vi "DSP_conditioning_Tx.vi"(1 "reset":bool, 4 "tx.frequency shift":fxp<+/-,48,0>, 5 "IQ data":T1, 6 "tx.phase":fxp<+/-,21,0>, 7 "input valid":bool, 8 "tx.delay":fxp<+/-,18,0>, 9 "tx.impairments":T3, 10 "tx.input sample rate":fxp<+,48,1>, 11 "tx.gain":T2) -> (0 "tx.dsp reset done":bool, 2 "output valid":bool, 3 "data out":T1)   [LabVIEW 2017]
uses:
  <instrlib>/_niInstr/DSP/v1/Shared/Public/IQ Impairments.ctl
  <instrlib>/_niInstr/DSP/v1/Shared/Public/IQ Gain.ctl
  <instrlib>/_niInstr/DSP/v1/Shared/Public/IQ Data.ctl
  <instrlib>/_niInstr/DSP/v1/FPGA/Public/Sub VIs/Digital Gain/Digital Gain - 1 spc.vi
  <instrlib>/_niInstr/DSP/v1/FPGA/Public/Sub VIs/Frequency Shift/Frequency Shift - 1 spc.vi
  <instrlib>/_niInstr/DSP/v1/FPGA/Public/Sub VIs/IQ Impairments/IQ Impairments - 1 spc.vi
  <instrlib>/_niInstr/DSP/v1/FPGA/niInstr DSP v1 FPGA.lvlib
  <instrlib>/_niInstr/Basic Elements/v1/FPGA/niInstr Basic Elements v1 FPGA.lvlib
  <instrlib>/_niInstr/DSP/v1/FPGA/Public/Sub VIs/Fractional Interpolator/Fractional Interpolator - 1 spc - 2x oc.vi
  <instrlib>/_niInstr/DSP/v1/Shared/niInstr DSP v1 Shared.lvlib
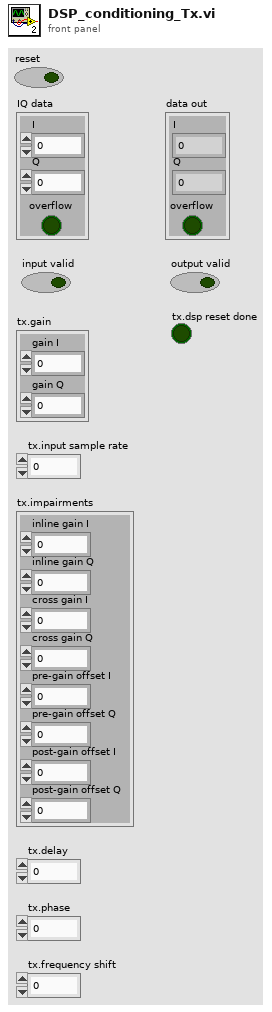
[diagram p1: front panel]
types:
  T1 = typedef "niInstr DSP v1 Shared.lvlib/IQ Data.ctl" = cluster{"I":fxp<+/-,18,1>, "Q":fxp<+/-,18,1>, "overflow":bool}
  T2 = typedef "niInstr DSP v1 Shared.lvlib/IQ Gain.ctl" = cluster{"gain I":fxp<+/-,24,3>, "gain Q":fxp<+/-,24,3>}
  T3 = typedef "niInstr DSP v1 Shared.lvlib/IQ Impairments.ctl" = cluster{"inline gain I":fxp<+/-,18,1>, "inline gain Q":fxp<+/-,18,1>, "cross gain I":fxp<+/-,18,1>, "cross gain Q":fxp<+/-,18,1>, "pre-gain offset I":fxp<+/-,18,1>, "pre-gain offset Q":fxp<+/-,18,1>, "post-gain offset I":fxp<+/-,18,1>, "post-gain offset Q":fxp<+/-,18,1>}
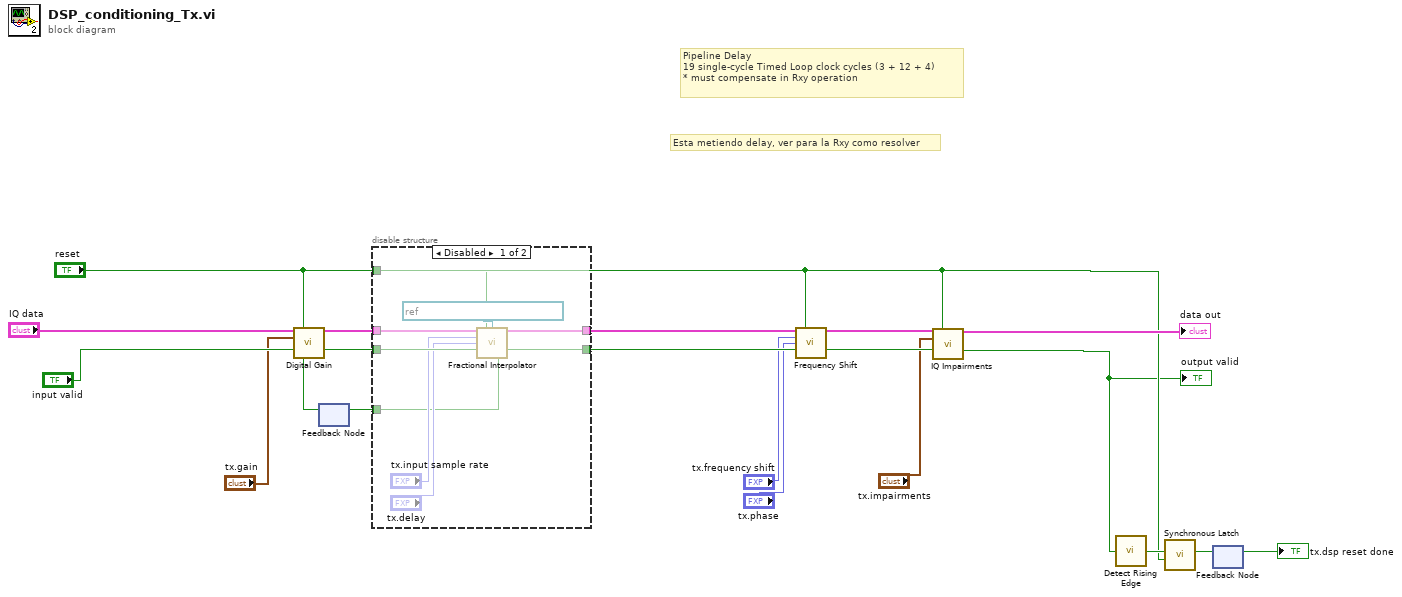
[diagram p0: block diagram]
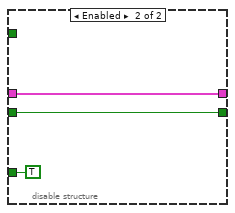
[diagram p2: hidden frame]
diagram:
  # "Pipeline Delay \n19 single-cycle Timed Loop clock cycles (3 + 12 + 4)\n* must compensate in Rxy operation"
  # "Esta metiendo delay, ver para la Rxy como resolver"
  n1 = feedback #1() -> (w6:bool)  [unwired: 1 in]
  n2 = call-poly <instrlib>:"Digital Gain.vi"("data in"="IQ data", "reset"="reset", "gain"="tx.gain", "input valid"="input valid", "ready for output (T)"=w6) -> ("data out"=w7:T1, "output valid"=w8:bool)  [unwired: 8 in, 1 out]
  n3 = disable-structure shown="Disabled" {
    disable-tunnel: [w29 w31] -> w10
    disable-tunnel: [w28 w32] -> w9
    disable-tunnel: w8 -> [w26 w31]
    disable-tunnel: w7 -> [w23 w32]
    disable-tunnel: "reset" -> [w22 _]
    disable-tunnel: [w21 TRUE ("signal")] -> w1
    frame Disabled {
      n4 = call-poly <instrlib>:"Fractional Interpolator.vi"("data in"=w23, "reset"=w22, "clock x 2"=refnum<k21> "IO Module\\Data Clock x2", "input sample rate"="tx.input sample rate", "delay"="tx.delay", "input valid"=w26) -> ("data out"=w28:T1, "output valid"=w29:bool, "ready for input"=w21:bool)  [unwired: 6 in, 1 out]
    }
    frame Enabled {
    }
  }
  n5 = feedback-in #1(w1) -> ()
  n6 = call-poly <instrlib>:"Frequency Shift.vi"("data in"=w9, "reset"="reset", "frequency shift"="tx.frequency shift", "phase"="tx.phase", "input valid"=w10) -> ("data out"=w11:T1, "output valid"=w12:bool)  [unwired: 8 in, 1 out]
  n7 = call-poly <instrlib>:"IQ Impairments.vi"("data in"=w11, "reset"="reset", "impairments"="tx.impairments", "input valid"=w12) -> ("data out"=→"data out":T1, "output valid"=w13:bool)  [unwired: 9 in, 1 out]
  "output valid" <- w13
  n8 = call <instrlib>:"Detect Rising Edge.vi"("signal"=w13) -> ("edge detected"=w16:bool)  [unwired: 14 in]
  n9 = call <instrlib>:"Synchronous Latch.vi"("clear"="reset", "set"=w16) -> ("out"=w15:bool)  [unwired: 9 in]
  n10 = feedback #2() -> (→"tx.dsp reset done":bool)  [unwired: 1 in]
  n11 = feedback-in #2(w15) -> ()
